vi "Remove Bitfiles.vi"(8 "error in (no error)":errorcluster, 10 "RIO Addresses":string[](array[string]), 11 "Item Ref in":T1 format="%.0x") -> (0 "error out":errorcluster, 1 "Previous master":string, 2 "Need to select a new master?":bool, 3 "Item Ref out":T1 format="%.0x")   [LabVIEW 2017, in "Engine Simulation Toolkit System Explorer.lvlib"]
uses:
  Engine Simulation Toolkit System Explorer.lvlib
  <vilib>/NI Veristand/Custom Device API/Custom Device Item Ref.ctl
  Shared/Properties.vi
  <vilib>/NI Veristand/Custom Device API/Get Item Property (String Array).vi
  <userlib>/_OpenG.lib/array/array.llb/Filter 1D Array (String)__ogtk.vi
  <vilib>/NI Veristand/Custom Device API/Set Item Property (String Array).vi
  <vilib>/NI Veristand/Custom Device API/Get Item Property (String).vi
  <userlib>/_OpenG.lib/array/array.llb/Remove Duplicates from 1D Array (String)__ogtk.vi
  <vilib>/NI Veristand/Custom Device API/Custom Device API.lvlib
  Shared/Engine Simulation Toolkit Shared.lvlib
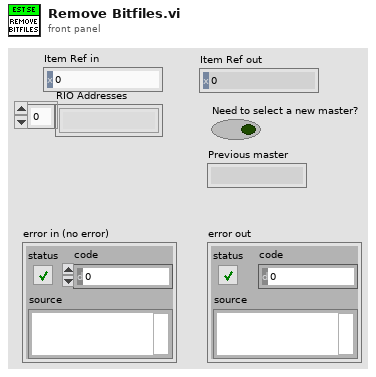
[diagram p1: front panel]
types:
  T1 = typedef "Custom Device API.lvlib/Custom Device Item Ref.ctl" = u64
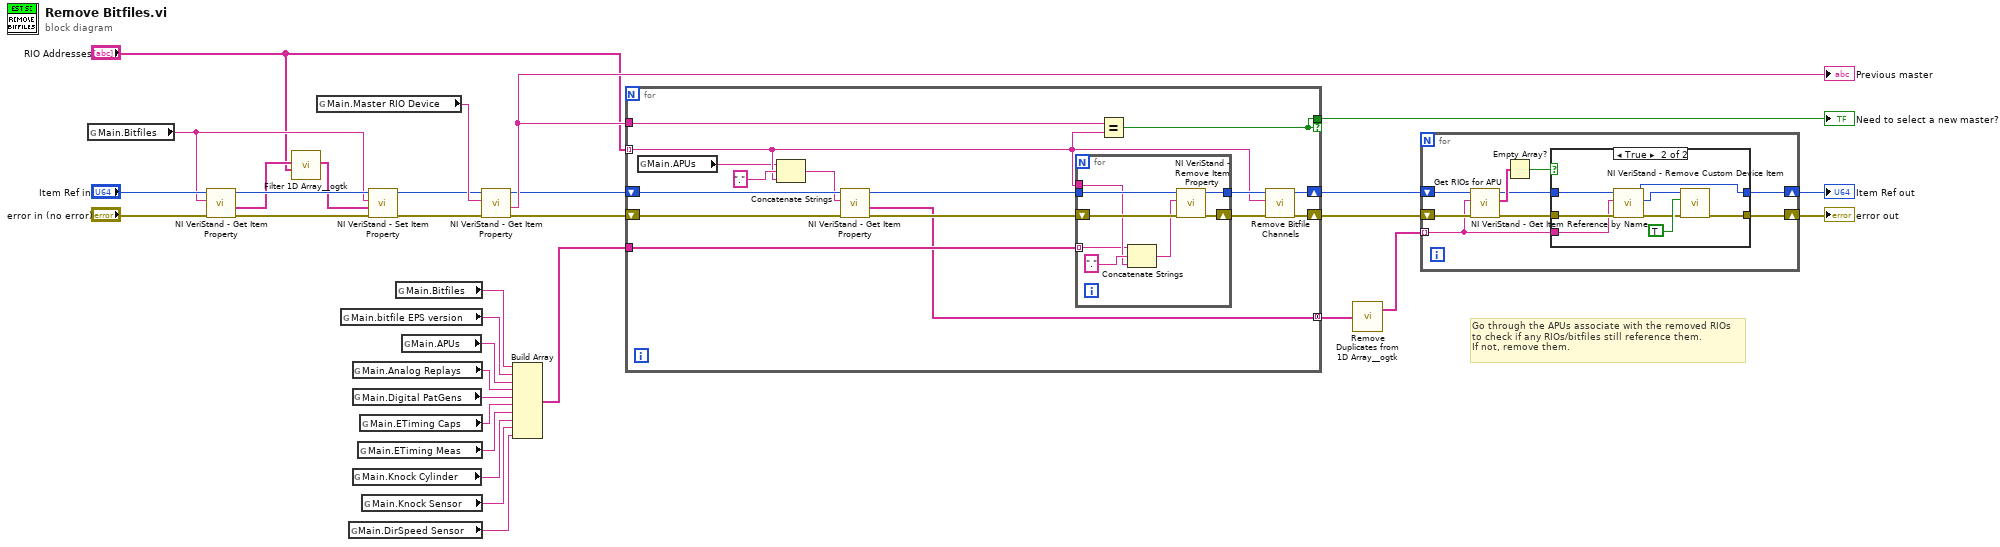
[diagram p0: block diagram]
diagram:
  # "Go through the APUs associate with the removed RIOs\nto check if any RIOs/bitfiles still reference them.\nIf not, remove them."
  n1 = global read "Properties.vi" "Main.Bitfiles"() -> (w9:string)
  n2 = call-poly <vilib>:"NI VeriStand - Get Item Property.vi"("error in (no error)"="error in (no error)", "Property Name"=w9, "Item Ref in"="Item Ref in") -> ("error out"=w14:errorcluster, "Value"=w10:string[], "Item Ref out"=w12:T1)  [unwired: 5 in, 1 out]
  n3 = call-poly <userlib>:"Filter 1D Array__ogtk.vi"("items to filter"="RIO Addresses", "array"=w10) -> ("filtered array"=w7:string[])  [unwired: 4 in, 1 out]
  n4 = global read "Properties.vi" "Main.Master RIO Device"() -> (w28:string)
  n5 = global read "Properties.vi" "Main.bitfile EPS version"() -> (w17:string)
  n6 = global read "Properties.vi" "Main.DirSpeed Sensor"() -> (w19:string)
  n7 = global read "Properties.vi" "Main.Analog Replays"() -> (w26:string)
  n8 = global read "Properties.vi" "Main.Digital PatGens"() -> (w25:string)
  n9 = global read "Properties.vi" "Main.Knock Cylinder"() -> (w21:string)
  n10 = global read "Properties.vi" "Main.ETiming Meas"() -> (w23:string)
  n11 = global read "Properties.vi" "Main.ETiming Caps"() -> (w24:string)
  n12 = global read "Properties.vi" "Main.Knock Sensor"() -> (w20:string)
  n13 = call-poly <vilib>:"NI VeriStand - Set Item Property.vi"("error in (no error)"=w14, "Value"=w7, "Property Name"=w9, "Item Ref in"=w12) -> ("error out"=w16:errorcluster, "Item Ref out"=w11:T1)  [unwired: 5 in, 1 out]
  n14 = global read "Properties.vi" "Main.Bitfiles"() -> (w18:string)
  n15 = global read "Properties.vi" "Main.APUs"() -> (w22:string)
  n16 = call-poly <vilib>:"NI VeriStand - Get Item Property.vi"("error in (no error)"=w16, "Property Name"=w28, "Item Ref in"=w11) -> ("error out"=w30:errorcluster, "Value"=w32:string, "Item Ref out"=w29:T1)  [unwired: 5 in, 1 out]
  "Previous master" <- w32
  n17 = Build Array(w18, w17, w22, w26, w25, w24, w23, w21, w20, w19) -> (w27:string[])
  n18 = for {
    shift-right: [w45] -> w3
    shift-left: w30 -> [w39]
    tunnel: w27 -> [w48]
    tunnel: w32 -> [w44]
    tunnel: [w43] -> w31 if=w43
    tunnel: "RIO Addresses" -> [w36] mode=indexing
    tunnel: [w33] -> w6 mode=concatenating
    shift-right: [w42] -> w4
    shift-left: w29 -> [w40]
    n19 = global read "Properties.vi" "Main.APUs"() -> (w35:string)
    n20 = Concatenate Strings(w35, "." ("string"), w36) -> (w34:string)
    n21 = call-poly <vilib>:"NI VeriStand - Get Item Property.vi"("error in (no error)"=w39, "Property Name"=w34, "Item Ref in"=w40) -> ("error out"=w38:errorcluster, "Value"=w33:string[], "Item Ref out"=w41:T1)  [unwired: 5 in, 1 out]
    n22 = for {
      tunnel: w41 -> [w55]
      tunnel: w36 -> [w52]
      shift-right: [w54] -> w47
      shift-left: w38 -> [w56]
      tunnel: w48 -> [w51] mode=indexing
      tunnel: [w49] -> w46
      n23 = Concatenate Strings(w51, "." ("string"), w52) -> (w50:string)
      n24 = call <vilib>:"NI VeriStand - Remove Item Property.vi"("error in (no error)"=w56, "Property Name"=w50, "Item Ref in"=w55) -> ("error out"=w54:errorcluster, "Item Ref out"=w49:T1)  [unwired: 6 in, 1 out]
    }
    n25 = Equal?(x=w44, y=w36) -> (x = y?=w43:bool)
    n26 = call "Remove Bitfile Channels.vi"("error in (no error)"=w47, "RIO name"=w36, "Item Ref in"=w46) -> ("error out"=w45:errorcluster, "Item Ref out"=w42:T1)  [unwired: 7 in]
  }
  "Need to select a new master?" <- w31
  n27 = call-poly <userlib>:"Remove Duplicates from 1D Array__ogtk.vi"("Input Array"=w6) -> ("Output Array"=w1:string[])  [unwired: 1 out]
  n28 = for {
    shift-right: [w58] -> w5
    shift-left: w4 -> [w65]
    shift-right: [w57] -> w2
    shift-left: w3 -> [w64]
    tunnel: w1 -> [w59] mode=indexing
    n29 = call "Get RIOs for APU.vi"("error in (no error)"=w64, "APU name"=w59, "Item Ref in"=w65) -> ("error out"=w60:errorcluster, "RIO Addresses"=w63:string[], "Item Ref out"=w61:T1)  [unwired: 6 in]
    n30 = Empty Array?(array=w63) -> (empty?=w62:bool)
    n31 = case shown="True" w62 {
      tunnel: w61 -> [w67 w75]
      tunnel: w60 -> [w66 w74]
      tunnel: w59 -> [_ w73]
      tunnel: [w67 w69] -> w58
      tunnel: [w66 w68] -> w57
      frame False {
      }
      frame True {
        n32 = call <vilib>:"NI VeriStand - Get Item Reference by Name.vi"("error in (no error)"=w74, "Item Name"=w73, "Parent Ref in"=w75) -> ("error out"=w71:errorcluster, "Item Ref"=w70:T1, "Parent Ref out"=w69:T1)  [unwired: 5 in, 1 out]
        n33 = call <vilib>:"NI VeriStand - Remove Custom Device Item.vi"("error in (no error)"=w71, "Force Delete (F)"=TRUE, "Item Ref in"=w70) -> ("error out"=w68:errorcluster)  [unwired: 7 in, 1 out]
      }
    }
  }
  "error out" <- w2
  "Item Ref out" <- w5
